vi "Read_From_Spreadsheet_2012.vi"(7 "My File has Row Headers":bool, 9 "precision (6)":i16, 11 "Spreadsheet path (.csv)":path=path "C:/Users/husmith/Desktop/MyData.csv") -> (2 "Data Dsiplay":dbl[][](array[numeric]), 3 "Spread Sheet Display":string[][](array[string]))   [LabVIEW 2025]
uses:
  <vilib>/Utility/file.llb/Read From Spreadsheet File (string).vi
  <vilib>/Utility/file.llb/Read From Spreadsheet File (DBL).vi
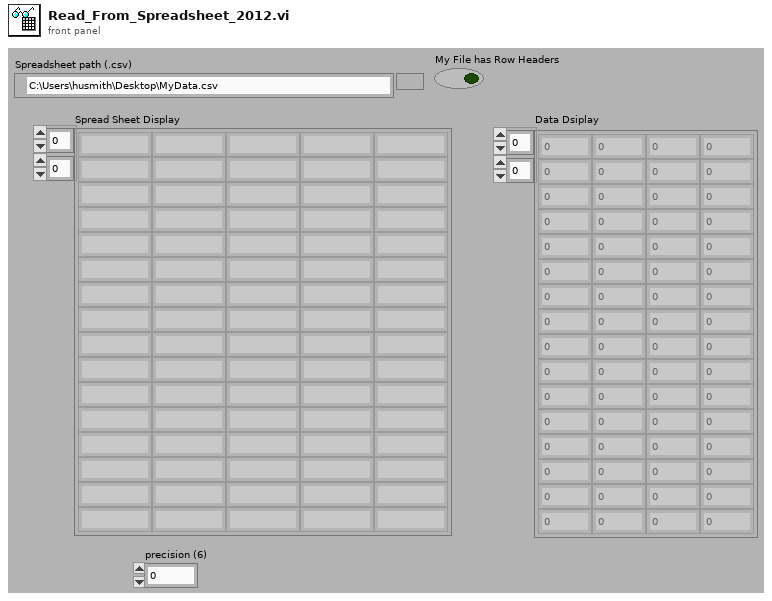
[diagram p1: front panel]
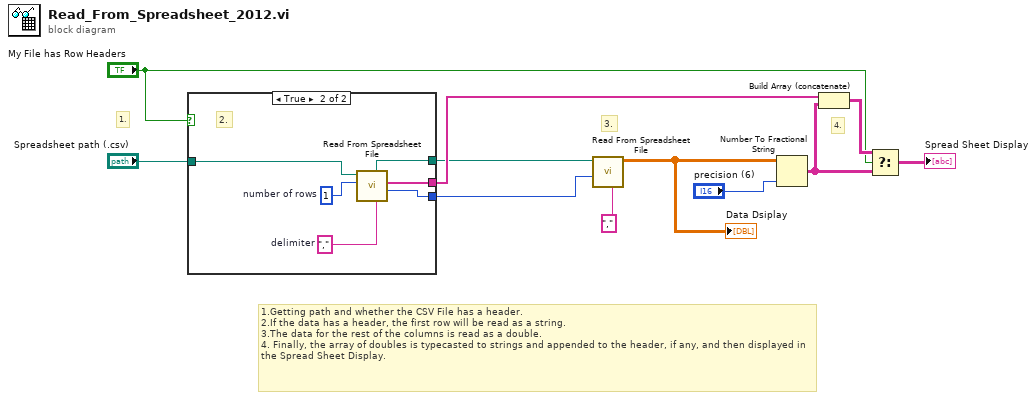
[diagram p0: block diagram]
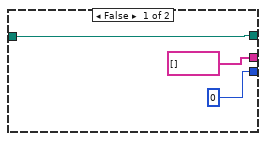
[diagram p2: hidden frame]
diagram:
  # "4."
  # "1.Getting path and whether the CSV File has a header.\n2.If the data has a header, the first row will be read as a string.\n3.The data for the rest of the columns is read as a double.\n4. Finally, the array of doubles is typecasted to strings and appended to the header, if any, and then displayed in the Spread Sheet Display."
  # "3."
  # "1."
  n1 = case shown="True" "My File has Row Headers" {
    tunnel: "Spreadsheet path (.csv)" -> [w12 w20]
    tunnel: [string[] [] ("first row") w18] -> w9
    tunnel: [0 ("mark after read (chars.)") w17] -> w4
    tunnel: [w12 w15] -> w8
    frame False {
    }
    frame True {
      w16 = 1  # number of rows
      w19 = ","  # delimiter
      # "2."
      n2 = call-poly <vilib>:"Read From Spreadsheet File.vi"("delimiter (\\t)"=w19, "number of rows (all:-1)"=w16, "file path (dialog if empty)"=w20) -> ("mark after read (chars.)"=w17:i32, "first row"=w18:string[], "new file path (Not A Path if cancelled)"=w15:path)  [unwired: 4 in, 2 out]
    }
  }
  n3 = call-poly <vilib>:"Read From Spreadsheet File.vi"("delimiter (\\t)"="," ("delimiter (\\t)"), "start of read offset (chars.:0)"=w4, "file path (dialog if empty)"=w8) -> ("all rows"=w2:dbl[][])  [unwired: 4 in, 4 out]
  "Data Dsiplay" <- w2
  n4 = Number To Fractional String(number=w2, precision (6)="precision (6)") -> (F-format string=w3:string[][])  [unwired: 2 in]
  n5 = Build Array (concatenate)(w9, w3) -> (w7:string[][])
  n6 = Select(t=w7, s="My File has Row Headers", f=w3) -> (s? t:f=→"Spread Sheet Display":string[][])
